vi "Boss5.vi"() -> ()   [LabVIEW 2017]
panel:
  out "?":bool
  in  "Boss":bool
  in  "Boolean 5":bool
  in  "Boolean 4":bool
  in  "Boolean 3":bool
  in  "2":bool
  in  "?":bool
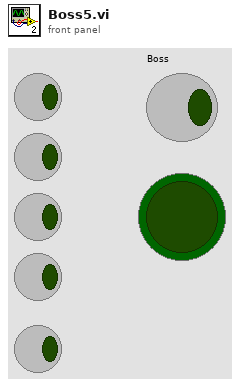
[diagram p1: front panel]
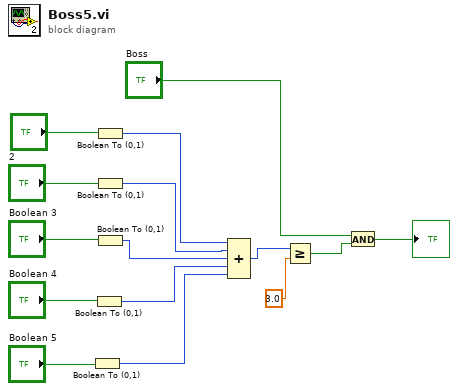
[diagram p0: block diagram]
diagram:
  n1 = Boolean To (0,1)(Boolean="Boolean 5") -> (0, 1=w11:i16)
  n2 = Boolean To (0,1)(Boolean="Boolean 4") -> (0, 1=w12:i16)
  n3 = Boolean To (0,1)(Boolean="?") -> (0, 1=w15:i16)
  n4 = Boolean To (0,1)(Boolean="2") -> (0, 1=w14:i16)
  n5 = Boolean To (0,1)(Boolean="Boolean 3") -> (0, 1=w13:i16)
  n6 = Compound Arithmetic op=ADD(w15, w14, w13, w12, w11) -> (w4:i16)
  n7 = Greater Or Equal?(x=w4, y=3.0) -> (x >= y?=w2:bool)
  n8 = And(x="Boss", y=w2) -> (x .and. y?=→"?":bool)
